vi "List.vi"(8 "error in (no error)":errorcluster, 11 "LUnit Test Suite In":refnum<class "LUnit Test Suite.lvclass">) -> (0 "error out":errorcluster, 2 "List of Runnables":string[](array[string]))   [LabVIEW 2020, in "LUnit Test Suite.lvclass"]
uses:
  LUnit Test Suite.lvclass
  LUnit Test Suite.lvclass/LUnit Test Suite.ctl
  Core/Runnable/Runnable.lvclass
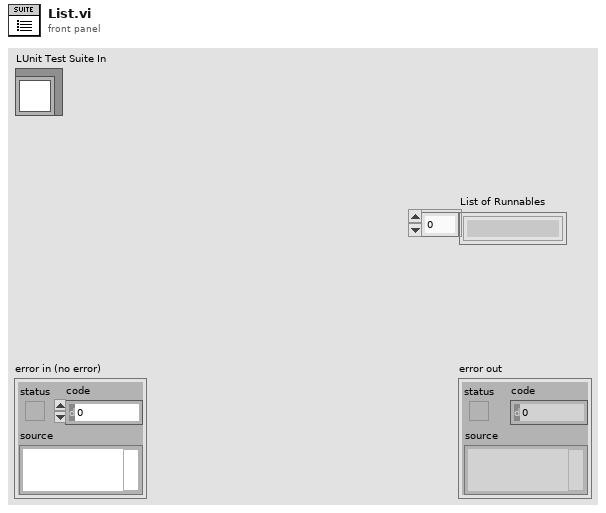
[diagram p1: front panel]
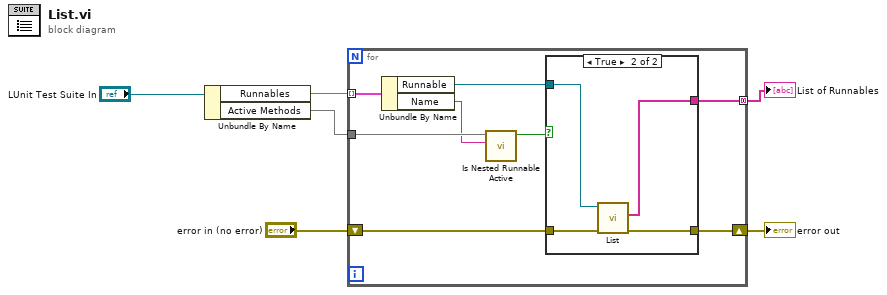
[diagram p0: block diagram]
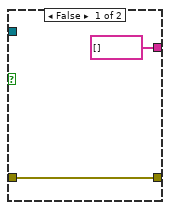
[diagram p2: hidden frame]
diagram:
  n1 = Unbundle By Name("LUnit Test Suite In") -> ("Runnables"=w5:map{string, refnum<class "Runnable.lvclass">}, "Active Methods"=w1:set{string})
  n2 = for {
    tunnel: w5 -> [w14] mode=indexing
    tunnel: [w12] -> w4 mode=concatenating
    shift-right: [w10] -> w2
    shift-left: "error in (no error)" -> [w11]
    tunnel: w1 -> [w9]
    n3 = Unbundle By Name(w14) -> ("Runnable"=w13:refnum<class "Runnable.lvclass">, "Name"=w8:string)
    n4 = call "Is Nested Runnable Active"("Name"=w8, "Active Methods"=w9) -> ("found?"=w7:bool)  [unwired: 9 in]
    n5 = case shown="True" w7 {
      tunnel: w13 -> [_ w20]
      tunnel: [string[] [] ("List of Runnables") w19] -> w12
      tunnel: w11 -> [w15 w18]
      tunnel: [w15 w17] -> w10
      frame False {
      }
      frame True {
        n6 = call-dynamic "List.vi"("error in (no error)"=w18, "Runnable In"=w20) -> ("error out"=w17:errorcluster, "List of Runnables"=w19:string[])  [unwired: 8 in]
      }
    }
  }
  "error out" <- w2
  "List of Runnables" <- w4
